vi "Switch Read.vi"(8 "error in (no error)":errorcluster, 11 "HG_LIB in":T1) -> (0 "error out":errorcluster, 1 "Limit L":bool, 2 "Limit H":bool, 3 "HG_LIB out":T2)   [LabVIEW 2020]
uses:
  <vilib>/High Genius/HG_WSI_Tookit/Dependencies/Library/Digital Input and Output/Digital Input and Output.lvclass
  C:/Program Files (x86)/National Instruments/LabVIEW 2020/vi.lib/High Genius/HG_WSI_Tookit/Dependencies/Library/HG_LIB/HG_LIB.lvclass
  <vilib>/High Genius/HG_WSI_Tookit/Dependencies/Library/HG_LIB/HG_LIB.lvclass/HG_LIB.ctl
  <vilib>/High Genius/HG_WSI_Tookit/Dependencies/Library/HG_LIB/HG_LIB.lvclass
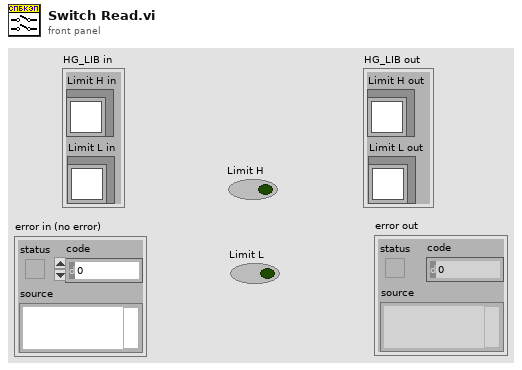
[diagram p1: front panel]
types:
  T1 = cluster{"Limit H in":refnum<class "Digital Input and Output.lvclass">, "Limit L in":refnum<class "Digital Input and Output.lvclass">}
  T2 = cluster{"Limit H out":refnum<class "Digital Input and Output.lvclass">, "Limit L out":refnum<class "Digital Input and Output.lvclass">}
  T3 = cluster{"data":cluster{"ai22":sgl, "ai23":sgl, "ai24":sgl, "ai25":sgl, "pulse12":i32, "pulse13":i32, "pwm14":i32, "pwm15":i32, "pwm16":i32, "do17":bool, "do18":bool, "do19":bool, "do20":bool, "do21":bool, "di11":bool, "di9":bool, "motor0":u8, "motor1":u8, "motor2":u8, "motor3":u8, "dir00":u8, "dir01":u8, "dir02":u8, "dir03":u8, "dir10":u8, "dir11":u8, "dir12":u8, "dir13":u8, "limit0":bool, "limit1":bool, "limit2":bool, "limit3":bool, "limit4":bool, "limit5":bool, "limit6":bool, "limit7":bool, "lsb0H":u8, "lsb1H":u8, "lsb2H":u8, "lsb3H":u8, "lsb0L":u8, "lsb1L":u8, "lsb2L":u8, "lsb3L":u8, "enc0_counters":u32, "enc1_counters":u32, "enc2_counters":u32, "enc3_counters":u32, "counter10":u32, "counter8":u32, "reset_enc0":bool, "reset_enc1":bool, "reset_enc2":bool, "reset_enc3":bool, "pitch":sgl, "roll":sgl, "yaw":sgl, "zero_yaw":bool}}
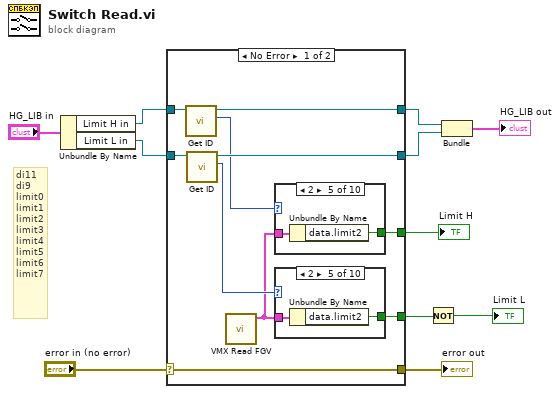
[diagram p0: block diagram]
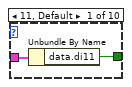
[diagram p2: hidden frame]
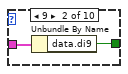
[diagram p3: hidden frame]
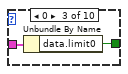
[diagram p4: hidden frame]
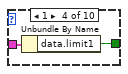
[diagram p5: hidden frame]
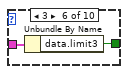
[diagram p6: hidden frame]
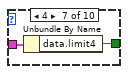
[diagram p7: hidden frame]
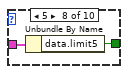
[diagram p8: hidden frame]
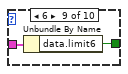
[diagram p9: hidden frame]
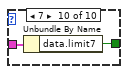
[diagram p10: hidden frame]
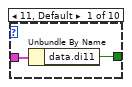
[diagram p11: hidden frame]
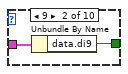
[diagram p12: hidden frame]
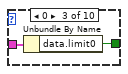
[diagram p13: hidden frame]
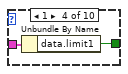
[diagram p14: hidden frame]
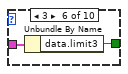
[diagram p15: hidden frame]
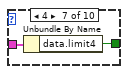
[diagram p16: hidden frame]
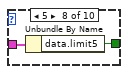
[diagram p17: hidden frame]
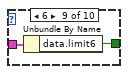
[diagram p18: hidden frame]
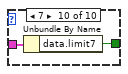
[diagram p19: hidden frame]
diagram:
  # "di11\ndi9\nlimit0\nlimit1\nlimit2\nlimit3\nlimit4\nlimit5\nlimit6\nlimit7"
  n1 = Unbundle By Name("HG_LIB in") -> ("Limit H in"=w4:refnum<class "Digital Input and Output.lvclass">, "Limit L in"=w3:refnum<class "Digital Input and Output.lvclass">)
  n2 = case shown="No Error" "error in (no error)" {
    selector: "error in (no error)" -> [w17 w64]
    tunnel: [w17 w64] -> w10
    tunnel: [w20 w63] -> w8
    tunnel: w3 -> [w21 w63]
    tunnel: [w18 _] -> w2
    tunnel: w4 -> [w16 w62]
    tunnel: [w14 w62] -> w9
    tunnel: [w12 _] -> w6
    frame No Error {
      n3 = call <vilib>:"Get ID.vi"("HG_LIB in"=w16) -> ("ID"=w15:u32, "HG_LIB out"=w14:refnum<class "Digital Input and Output.lvclass">)  [unwired: 9 in]
      n4 = call <vilib>:"Get ID.vi"("HG_LIB in"=w21) -> ("ID"=w19:u32, "HG_LIB out"=w20:refnum<class "Digital Input and Output.lvclass">)  [unwired: 9 in]
      n5 = call <vilib>:"VMX Read FGV.vi"() -> ("Read Data"=w13:T3)  [unwired: 10 in, 1 out]
      n6 = case shown="2" w15 {
        tunnel: w13 -> [w23 w25 w26 w29 w30 w33 w35 w37 w39 w41]
        tunnel: [w22 w24 w27 w28 w31 w32 w34 w36 w38 w40] -> w12
        frame 11, Default {
          n7 = Unbundle By Name(w23) -> ("data.di11"=w22:bool)
        }
        frame 9 {
          n8 = Unbundle By Name(w25) -> ("data.di9"=w24:bool)
        }
        frame 0 {
          n9 = Unbundle By Name(w26) -> ("data.limit0"=w27:bool)
        }
        frame 1 {
          n10 = Unbundle By Name(w29) -> ("data.limit1"=w28:bool)
        }
        frame 2 {
          n11 = Unbundle By Name(w30) -> ("data.limit2"=w31:bool)
        }
        frame 3 {
          n12 = Unbundle By Name(w33) -> ("data.limit3"=w32:bool)
        }
        frame 4 {
          n13 = Unbundle By Name(w35) -> ("data.limit4"=w34:bool)
        }
        frame 5 {
          n14 = Unbundle By Name(w37) -> ("data.limit5"=w36:bool)
        }
        frame 6 {
          n15 = Unbundle By Name(w39) -> ("data.limit6"=w38:bool)
        }
        frame 7 {
          n16 = Unbundle By Name(w41) -> ("data.limit7"=w40:bool)
        }
      }
      n17 = case shown="2" w19 {
        tunnel: w13 -> [w43 w45 w46 w49 w50 w53 w55 w57 w59 w61]
        tunnel: [w42 w44 w47 w48 w51 w52 w54 w56 w58 w60] -> w18
        frame 11, Default {
          n18 = Unbundle By Name(w43) -> ("data.di11"=w42:bool)
        }
        frame 9 {
          n19 = Unbundle By Name(w45) -> ("data.di9"=w44:bool)
        }
        frame 0 {
          n20 = Unbundle By Name(w46) -> ("data.limit0"=w47:bool)
        }
        frame 1 {
          n21 = Unbundle By Name(w49) -> ("data.limit1"=w48:bool)
        }
        frame 2 {
          n22 = Unbundle By Name(w50) -> ("data.limit2"=w51:bool)
        }
        frame 3 {
          n23 = Unbundle By Name(w53) -> ("data.limit3"=w52:bool)
        }
        frame 4 {
          n24 = Unbundle By Name(w55) -> ("data.limit4"=w54:bool)
        }
        frame 5 {
          n25 = Unbundle By Name(w57) -> ("data.limit5"=w56:bool)
        }
        frame 6 {
          n26 = Unbundle By Name(w59) -> ("data.limit6"=w58:bool)
        }
        frame 7 {
          n27 = Unbundle By Name(w61) -> ("data.limit7"=w60:bool)
        }
      }
    }
    frame Error {
    }
  }
  "error out" <- w10
  "Limit H" <- w6
  n28 = Not(x=w2) -> (.not. x?=→"Limit L":bool)
  n29 = Bundle("Limit H in"=w9, "Limit L in"=w8) -> (→"HG_LIB out":T1)  [unwired: 1 in]
